vi "Level.vi"(11 "DataIn":T1) -> (3 "DataOut":T1)   [LabVIEW 2018]
uses:
  controls/DataIn.ctl
  MatchDataClasses/MatchData/MatchData.lvclass
  controls/Tabuleiro.ctl
  controls/GameOption.ctl
  controls/Table.ctl
panel:
  in  "Sair":bool
  in  "Multiplayer - local":bool
  in  "Difícil":bool
  in  "Médio":bool
  in  "Fácil":bool
  # "Escolha o modo de jogo"
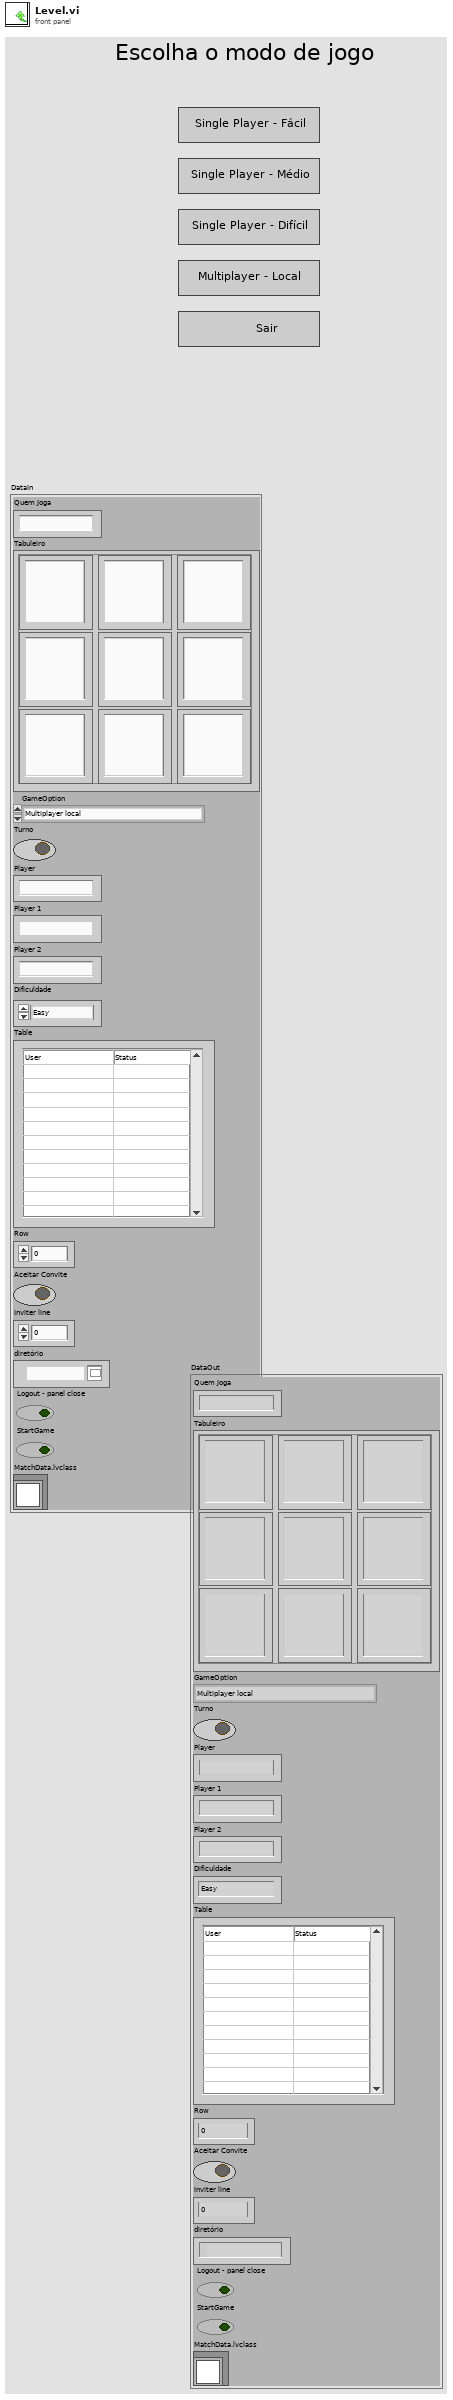
[diagram p1: front panel]
types:
  T1 = typedef "DataIn.ctl" = cluster{"Quem Joga":string, "Tabuleiro":T2, "GameOption":T3, "Turno":bool, "Player":string, "Player 1":string, "Player 2":string, "Dificuldade":enum16{"Easy", "Medium", "Hard"}, "Table":T4, "Row":u32, "Aceitar Convite":bool, "Inviter line":u32, "diretório":path, "Logout - panel close":bool, "StartGame":bool, "MatchData.lvclass":refnum<class "MatchData.lvclass">}
  T2 = typedef "Tabuleiro.ctl" = cluster{"(0,0)":string, "(1,0)":string, "(0,1)":string, "(1,1)":string, "(2,0)":string, "(1,2)":string, "(2,2)":string, "(0,2)":string, "(2,1) ":string}
  T3 = typedef "GameOption.ctl" = enum16{"Multiplayer local", "Multiplayer remoto", "Single Player", "Wait for Event", "Initialize", "Stop"}
  T4 = typedef "Table.ctl" = string[][]
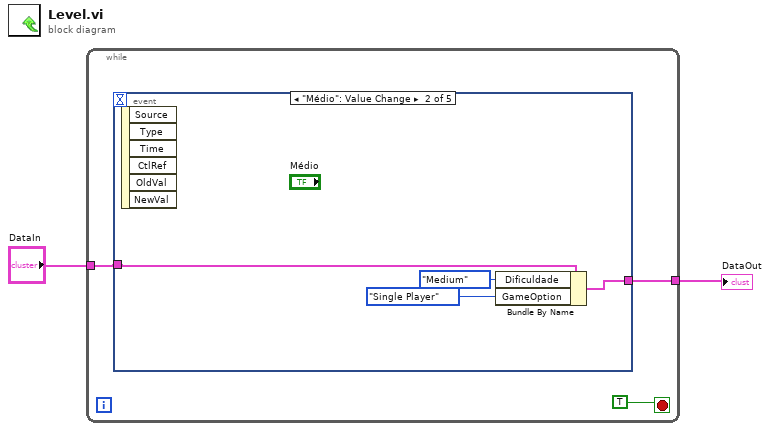
[diagram p0: block diagram]
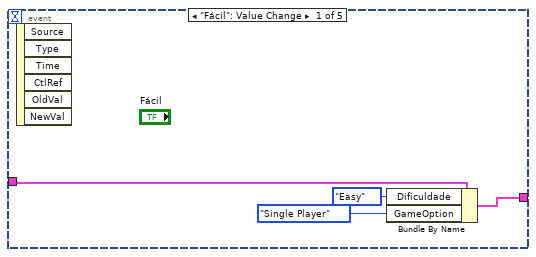
[diagram p2: hidden frame]
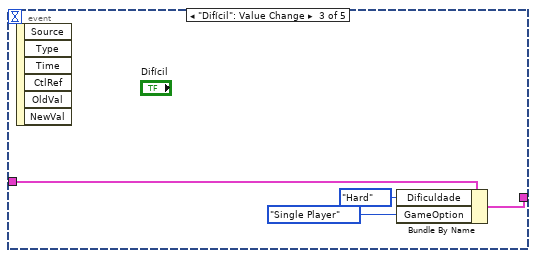
[diagram p3: hidden frame]
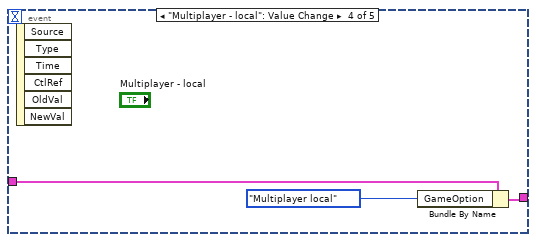
[diagram p4: hidden frame]
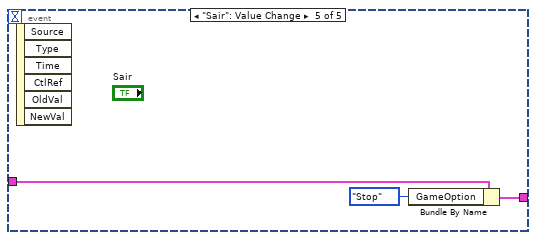
[diagram p5: hidden frame]
diagram:
  n1 = while {
    tunnel: "DataIn" -> [w3]
    tunnel: [w4] -> w1
    stop <- TRUE stop-if-true
    n2 = event shown="[1] \"Médio\": Value Change" {
      selector: _ -> [_ _ _ _ _]
      dyn-events: _ -> [_ _ _ _ _]
      timeout: _ -> [_ _ _ _ _]
      tunnel: [w9 w13 w17 w20 w23] -> w4
      tunnel: w3 -> [w7 w11 w16 w19 w22]
      event "Fácil": Value Change {
        n3 = event-data() -> ()  [unwired: 1 in, 6 out]
        n4 = Bundle By Name(cluster=w7, "Dificuldade"=enum16{"Easy", "Medium", "Hard"}."Easy", "GameOption"=GameOption."Single Player") -> (w9:T1)
      }
      event "Médio": Value Change {
        n5 = event-data() -> ()  [unwired: 1 in, 6 out]
        n6 = Bundle By Name(cluster=w11, "Dificuldade"=enum16{"Easy", "Medium", "Hard"}."Medium", "GameOption"=GameOption."Single Player") -> (w13:T1)
      }
      event "Difícil": Value Change {
        n7 = event-data() -> ()  [unwired: 1 in, 6 out]
        n8 = Bundle By Name(cluster=w16, "Dificuldade"=enum16{"Easy", "Medium", "Hard"}."Hard", "GameOption"=GameOption."Single Player") -> (w17:T1)
      }
      event "Multiplayer - local": Value Change {
        n9 = event-data() -> ()  [unwired: 1 in, 6 out]
        n10 = Bundle By Name(cluster=w19, "GameOption"=GameOption."Multiplayer local") -> (w20:T1)
      }
      event "Sair": Value Change {
        n11 = event-data() -> ()  [unwired: 1 in, 6 out]
        n12 = Bundle By Name(cluster=w22, "GameOption"=GameOption."Stop") -> (w23:T1)
      }
    }
  }
  "DataOut" <- w1
